vi "SubPnl Load Check.vi"(8 "에러 입력":errorcluster caption="에러 입력(에러 없음)", 11 "VI참조":refnum<vi>[](array[refnum])) -> (0 "에러 출력":errorcluster, 3 "SPEC error?":bool)   [LabVIEW 2020]
uses:
  Variables/Global_Cal Info.vi
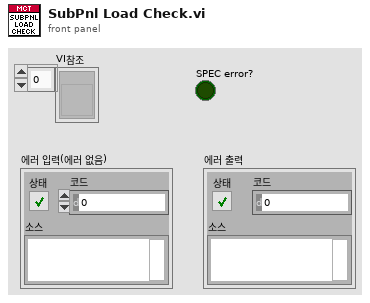
[diagram p1: front panel]
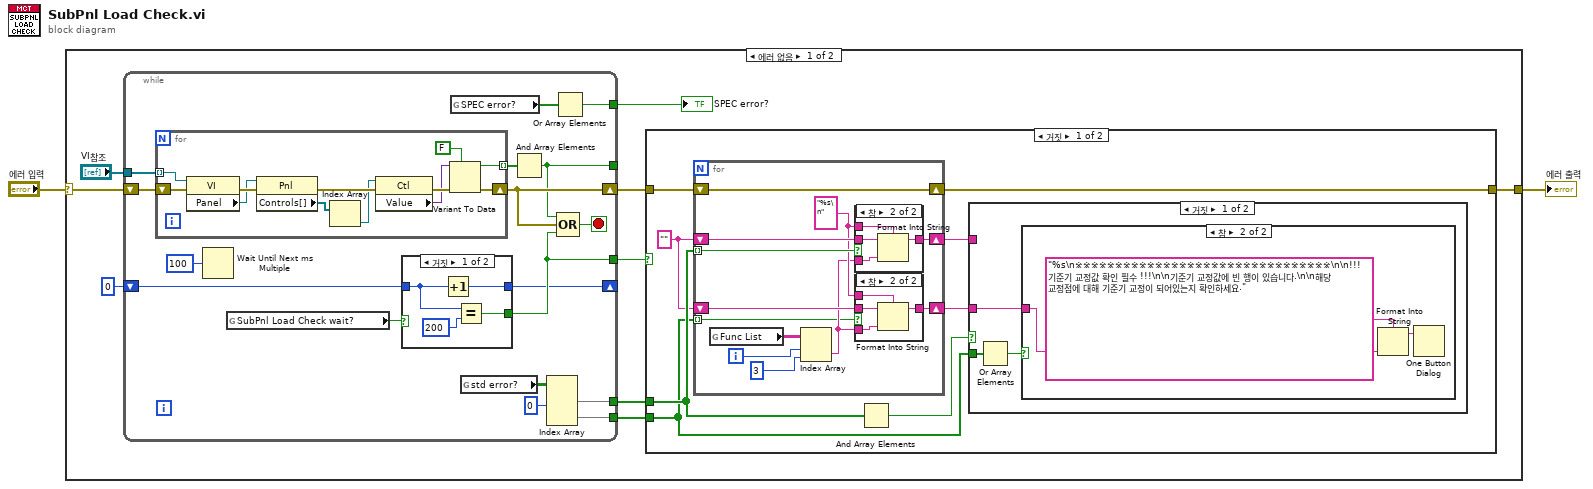
[diagram p0: block diagram]
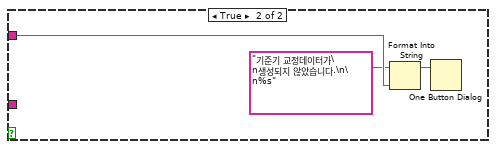
[diagram p5: hidden frame]
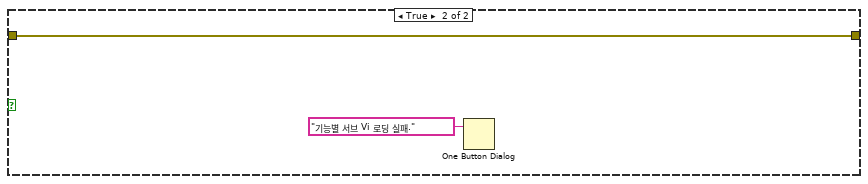
[diagram p6: hidden frame]
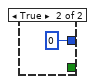
[diagram p7: hidden frame]
diagram:
  n1 = case shown="에러 없음" "에러 입력" {
    selector: "에러 입력" -> [w7 w87]
    tunnel: [w8 w87] -> w2
    frame No Error {
      n2 = while {
        shift-right: [w59] -> w11
        shift-left: w7 -> [w61]
        tunnel: [w65] -> w10
        tunnel: [w64] -> w9
        tunnel: [w63] -> w6
        tunnel: "VI참조" -> [w62]
        tunnel: [w58] -> _
        tunnel: [w56] -> w4
        shift-right: [w54] -> _
        shift-left: 0 -> [w53]
        stop <- w68 stop-if-true
        n3 = for {
          tunnel: w62 -> [w86] mode=indexing
          shift-right: [w78] -> w59
          shift-left: w61 -> [w85]
          tunnel: [w75] -> w60 mode=indexing
          n4 = property class="VI"(reference=w86, error in=w85) -> (error out=w84:errorcluster, "Panel"=w83:refnum<vi>)  [unwired: 1 out]
          n5 = property class="Pnl"(reference=w83, error in=w84) -> (error out=w81:errorcluster, "Controls[]"=w82:refnum<vi>[])  [unwired: 1 out]
          n6 = Index Array(array=w82) -> (element=w80:refnum<vi>)  [unwired: 1 in]
          n7 = property class="Ctl"(reference=w80, error in=w81) -> (error out=w79:errorcluster, "Value"=w77:variant)  [unwired: 1 out]
          n8 = Variant To Data(error in=w79, type=FALSE, Variant=w77) -> (data=w75:bool, error out=w78:errorcluster)
        }
        n9 = Wait Until Next ms Multiple(millisecond multiple=u32 100 ("ms 배수")) -> ()  [unwired: 1 out]
        n10 = global read "Global_Cal Info.vi" "SubPnl Load Check wait?"() -> (w55:bool)
        n11 = case shown="거짓" w55 {
          tunnel: [w72 _] -> w63
          tunnel: [w71 0] -> w54
          tunnel: w53 -> [w70 _]
          frame False {
            n12 = Increment(x=w70) -> (x+1=w71:i32)
            n13 = Equal?(x=w70, y=200) -> (x = y?=w72:bool)
          }
          frame True {
          }
        }
        n14 = global read "Global_Cal Info.vi" "SPEC error?"() -> (w57:bool[])
        n15 = global read "Global_Cal Info.vi" "std error?"() -> (w66:bool[][])
        n16 = And Array Elements(Boolean array=w60) -> (logical AND=w58:bool)
        n17 = Index Array(array=w66, index (col) #1=0 ("비활성화된 인덱스 (열)")) -> (element #1=w65:bool[], element #2=w64:bool[])  [unwired: 3 in]
        n18 = Or Array Elements(Boolean array=w57) -> (logical OR=w56:bool)
        n19 = Compound Arithmetic op=OR(w58, w59, w63) -> (w68:bool)
      }
      "SPEC error?" <- w4
      n20 = case shown="거짓" w6 {
        tunnel: w11 -> [w18 w52]
        tunnel: w10 -> [w17 _]
        tunnel: w9 -> [w16 _]
        tunnel: [w15 w52] -> w8
        frame False {
          w12 = ""
          n21 = for {
            shift-right: [w31] -> w15
            shift-left: w18 -> [w31]
            tunnel: w17 -> [w25] mode=indexing
            tunnel: w16 -> [w20] mode=indexing
            shift-right: [w26] -> w14
            shift-left: w12 -> [w27]
            shift-right: [w24] -> w13
            shift-left: w12 -> [w22]
            i -> [w28]
            w23 = "%s\n" ("포맷 문자열")
            n22 = global read "Global_Cal Info.vi" "Func List"() -> (w30:string[][])
            n23 = Index Array(array=w30, index (row)=w28, index (col)=3 ("비활성화된 인덱스 (열)")) -> (element=w21:string)
            n24 = case shown="참" w25 {
              tunnel: w27 -> [w37 w41]
              tunnel: [w37 w40] -> w26
              tunnel: w21 -> [_ w39]
              tunnel: w23 -> [_ w38]
              frame False {
              }
              frame True {
                n25 = Format Into String(format string=w38, initial string=w41, w39) -> (resulting string=w40:string)  [unwired: 1 in, 1 out]
              }
            }
            n26 = case shown="참" w20 {
              tunnel: w22 -> [w32 w36]
              tunnel: [w32 w35] -> w24
              tunnel: w21 -> [_ w34]
              tunnel: w23 -> [_ w33]
              frame False {
              }
              frame True {
                n27 = Format Into String(format string=w33, initial string=w36, w34) -> (resulting string=w35:string)  [unwired: 1 in, 1 out]
              }
            }
          }
          n28 = And Array Elements(Boolean array=w17) -> (logical AND=w19:bool)
          n29 = case shown="거짓" w19 {
            tunnel: w14 -> [_ w50]
            tunnel: w16 -> [w43 _]
            tunnel: w13 -> [w42 _]
            frame False {
              n30 = Or Array Elements(Boolean array=w43) -> (logical OR=w44:bool)
              n31 = case shown="참" w44 {
                tunnel: w42 -> [_ w47]
                frame False {
                }
                frame True {
                  n32 = Format Into String(format string="%s\n※※※※※※※※※※※※※※※※※※※※※※※※※※※※※※※※\n\n!!! 기준기 교정값 확인 필수 !!!\n\n기준기 교정값에 빈 행이 있습니다.\n\n해당 교정점에 대해 기준기 교정이 되어있는지 확인하세요." ("포맷 문자열"), w47) -> (resulting string=w46:string)  [unwired: 2 in, 1 out]
                  n33 = One Button Dialog(message=w46) -> ()  [unwired: 1 in, 1 out]
                }
              }
            }
            frame True {
              n34 = Format Into String(format string="기준기 교정데이터가\n생성되지 않았습니다.\n\n%s" ("포맷 문자열"), w50) -> (resulting string=w48:string)  [unwired: 2 in, 1 out]
              n35 = One Button Dialog(message=w48) -> ()  [unwired: 1 in, 1 out]
            }
          }
        }
        frame True {
          n36 = One Button Dialog(message="기능별 서브 Vi 로딩 실패." ("메시지")) -> ()  [unwired: 1 in, 1 out]
        }
      }
    }
    frame Error {
    }
  }
  "에러 출력" <- w2
